vi "Correlation Analysis.vi"() -> ()   [LabVIEW 2023]
doc: "This example shows how to compute the autocorrelation and crosscorrelation of a univariate time series with the TSA Auto-correlation Function VI and the TSA Cross-correlation Function VI respectively.\n\n<b>Instructions:</b>\n1) Run this VI.\n2) Change the delay between series 1 and series 2.\n3) Observe their cross-correlation."
uses:
  <vilib>/Waveform/WDTOps.llb/WDT Get Waveform Subset DBL (LV80).vi
  <vilib>/addons/Time Series Analysis/Correlation and Spectral Analysis.llb/TSA Cross-Correlation Function (Waveform).vi
  <vilib>/addons/Time Series Analysis/Correlation and Spectral Analysis.llb/TSA Auto-Correlation Function (Waveform).vi
  <vilib>/addons/_Advanced Signal Processing/NI_AdvSigProcTSA.lvlib
  <vilib>/measure/NI_MABase.lvlib
panel:
  in  "stop":bool
  in  "Positive Lag Only? (F)":bool
  out "Time Series":waveform(dbl)[](graph)
  in  "Delay between \nSeries 1 and 2":dbl=0.09999999999999996 min=0.0 max=0.2 step=0.01
  in  "Weighting 2":u16(ring) items=["biased (N)", "unbiased (N-k)"]
  out "Cross-Correlation between Series 1 and Series 2":cluster{"Ramp Pattern":dbl[], "Rxy":dbl[]}(graph)
  out "Auto-Correlation of Series 1":cluster{"Ramp Pattern":dbl[], "Rxy":dbl[]}(graph)
  in  "Weighting 1":u16(ring)=1 items=["biased (N)", "unbiased (N-k)"]
  # "Overview: Shows how to compute the autocorrelation and crosscorrelation of a univariate time series with the TSA Auto-Correlation Function VI and the TSA Cross-Correlation Function VI respectively.\nRequirements: LabVIEW Full Development System, Advanced Signal Processing Toolkit\nInstructions: \n1. Run this VI.\n2. Change the delay between series 1 and series 2.\n3. Observe their cross-correlation.\n4. Click Stop to stop the VI."
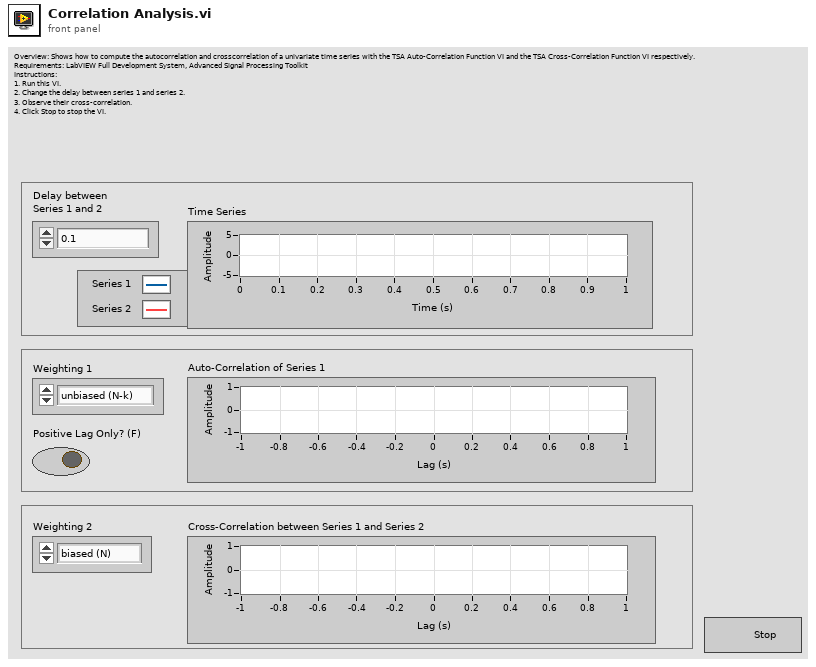
[diagram p1: front panel]
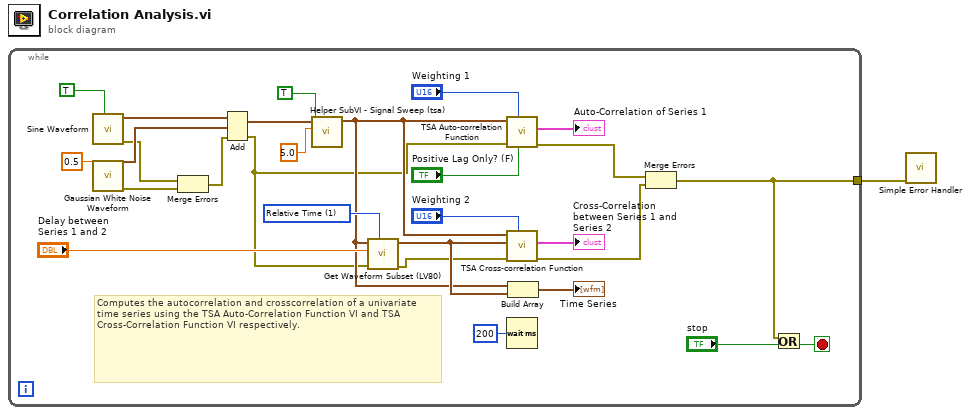
[diagram p0: block diagram]
diagram:
  n1 = while {
    tunnel: [w4] -> w1
    stop <- w17 stop-if-true
    w24 = u16 1 items=["Index", "Relative Time"] ("Mode")
    # "Computes the autocorrelation and crosscorrelation of a univariate time series using the TSA Auto-Correlation Function VI and TSA Cross-Correlation Function VI respectively."
    n2 = call <vilib>:"Sine Waveform.vi"("reset signal"=TRUE) -> ("error out"=w7:errorcluster, "signal out"=w13:waveform(dbl))  [unwired: 6 in, 3 out]
    n3 = call <vilib>:"Gaussian White Noise Waveform.vi"("standard deviation"=0.5) -> ("error out"=w6:errorcluster, "signal out"=w11:waveform(dbl))  [unwired: 4 in, 5 out]
    n4 = Merge Errors(w7, w6) -> (w3:errorcluster)
    n5 = Add(1:w11, 2:w13, 4:w3) -> (0:w12:waveform(dbl), 3:w2:errorcluster)
    n6 = call "Helper SubVI - Signal Sweep (tsa).vi"("reset"=TRUE, "shift (%)"=5.0, "Signal in"=w12) -> ("Signal out"=w15:waveform(dbl))  [unwired: 8 in]
    n7 = call-poly <vilib>:"Get Waveform Subset (LV80).vi"("start/duration format"=w24, "error in (no error)"=w2, "start samples/time"="Delay between \nSeries 1 and 2", "waveform in"=w15) -> ("error out"=w5:errorcluster, "waveform out"=w22:waveform(dbl))  [unwired: 1 in, 3 out]
    n8 = call-poly <vilib>:"TSA Auto-correlation Function.vi"("positive lag only? (F)"="Positive Lag Only? (F)", "weighting"="Weighting 1", "error in (no error)"=w2, "Xt"=w15) -> ("error out"=w20:errorcluster, "correlogram"=→"Auto-Correlation of Series 1":cluster{"Ramp Pattern":dbl[], "Rxy":dbl[]})  [unwired: 2 in, 4 out]
    n9 = call-poly <vilib>:"TSA Cross-correlation Function.vi"("weighting"="Weighting 2", "error in (no error)"=w5, "Yt"=w22, "Xt"=w15) -> ("error out"=w19:errorcluster, "correlogram"=→"Cross-Correlation between Series 1 and Series 2":cluster{"Ramp Pattern":dbl[], "Rxy":dbl[]})  [unwired: 1 in, 5 out]
    n10 = Wait (ms)(milliseconds to wait=u32 200 ("millisecond multiple")) -> ()  [unwired: 1 out]
    n11 = Build Array(w15, w22) -> (→"Time Series":waveform(dbl)[])
    n12 = Merge Errors(w20, w19) -> (w4:errorcluster)
    n13 = Or(x=w4, y="stop") -> (x .or. y?=w17:bool)
  }
  n14 = call <vilib>:"Simple Error Handler.vi"("error in (no error)"=w1) -> ()  [unwired: 1 in, 8 out]
